vi "Vision Align.vi"() -> (3 "YawOut":bool)   [LabVIEW 2019]
uses:
  <vilib>/Rock Robotics/WPI/ThirdParty/Sensors/navX/_TypeDefs/FRIC_navX_DeviceNumbersTypeDef.ctl
  <vilib>/Rock Robotics/Network Tables/NT Read Numeric Array.vi
  Driver Globals.vi
  <vilib>/Rock Robotics/Network Tables/NT Write Boolean.vi
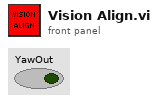
[diagram p1: front panel]
types:
  T1 = typedef "FRIC_navX_DeviceNumbersTypeDef.ctl" = enum16{"Dev0", "Dev1", "Dev2", "Dev3"}
  T2 = cluster{"Yaw":dbl, "Roll":dbl, "Pitch":dbl, "Heading":dbl, "Fused Heading":dbl}
  T3 = typedef "WPI_EncoderDevRef.ctl" = cluster{"DevStatus":errorcluster, "EncoderIndex":T4, "CounterIndex":T5, "DistancePerCount":dbl, "Decoding Type":T6}
  T4 = typedef "FPGA_EncoderIdx.ctl" = enum8{"Enc 0", "Enc 1", "Enc 2", "Enc 3", "Enc 4", "Enc 5", "Enc 6", "Enc 7", "Invalid"}
  T5 = typedef "FPGA_CounterCtrSystemIndex.ctl" = enum8{"Ctr 0", "Ctr 1", "Ctr 2", "Ctr 3", "Ctr 4", "Ctr 5", "Ctr 6", "Ctr 7", "Invalid"}
  T6 = typedef "WPI_EncoderType.ctl" = enum16{"1x", "2x", "4x"}
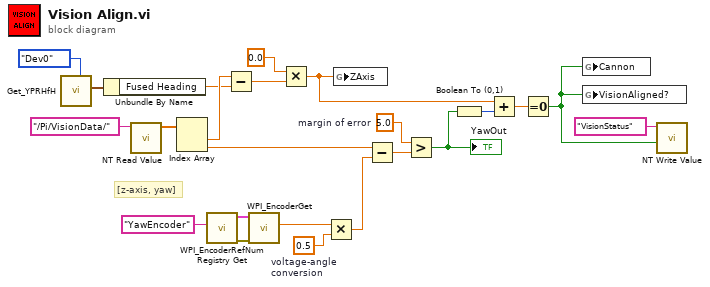
[diagram p0: block diagram]
diagram:
  w12 = 5.0  # margin of error
  w16 = 0.5  # voltage-angle conversion
  # "[z-axis, yaw]"
  n1 = call <vilib>:"Get_YPRHfH.vi"("Device Number"=FRIC_navX_DeviceNumbersTypeDef."Dev0") -> ("YRPHfH"=w9:T2)  [unwired: 10 in]
  n2 = Unbundle By Name(w9) -> ("Fused Heading"=w6:dbl)
  n3 = call-poly <vilib>:"NT Read Value.vi"("Name"="/Pi/VisionData/") -> ("Numeric Array"=w22:dbl[])  [unwired: 9 in, 1 out]
  n4 = Index Array(array=w22) -> (element #1=w7:dbl, element #2=w18:dbl)  [unwired: 2 in]
  n5 = call <vilib>:"WPI_EncoderRefNum Registry Get.vi"("refnum name"="YawEncoder") -> ("error out"=w20:errorcluster, "EncoderDevRef"=w21:T3)  [unwired: 9 in]
  n6 = Subtract(x=w7, y=w6) -> (x-y=w4:dbl)
  n7 = call <vilib>:"WPI_EncoderGet.vi"("error in (no error)"=w20, "EncoderDevRef"=w21) -> ("Distance"=w17:dbl)  [unwired: 4 in, 5 out]
  n8 = Multiply(x=0.0, y=w4) -> (x*y=w5:dbl)
  n9 = Multiply(x=w17, y=w16) -> (x*y=w15:dbl)
  n10 = global write "Driver Globals.vi" "ZAxis"(w5) -> ()
  n11 = Subtract(x=w18, y=w15) -> (x-y=w13:dbl)
  n12 = Greater?(x=w12, y=w13) -> (0:w1:bool)
  "YawOut" <- w1
  n13 = Boolean To (0,1)(Boolean=w1) -> (0, 1=w2:i16)
  n14 = Add(x=w5, y=w2) -> (x+y=w11:dbl)
  n15 = Equal To 0?(x=w11) -> (x = 0?=w10:bool)
  n16 = global write "Driver Globals.vi" "Cannon"(w10) -> ()
  n17 = global write "Driver Globals.vi" "VisionAligned?"(w10) -> ()
  n18 = call-poly <vilib>:"NT Write Value.vi"("Boolean"=w10, "Name"="VisionStatus") -> ()  [unwired: 9 in, 1 out]
